vi "level sensor(Sub-VI).vi"(11 "Tank C":dbl) -> (3 "Boolean":bool)   [LabVIEW 2020]
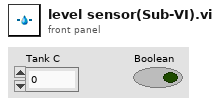
[diagram p1: front panel]
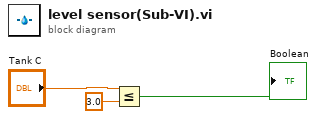
[diagram p0: block diagram]
diagram:
  n1 = Less Or Equal?(x="Tank C", y=3.0) -> (x <= y?=→"Boolean":bool)
